vi "Apply Direction.vi"(8 "error in (no error)":errorcluster, 11 "Tool Rectangle in":refnum<class "Tool Rectangle.lvclass">) -> (0 "error out":errorcluster, 3 "Tool Rectangle out":refnum<class "Tool Rectangle.lvclass">)   [LabVIEW 2019, in "Tool Rectangle.lvclass"]
uses:
  Tool Rectangle.lvclass
  Settings/ObjectSettings/ObjectSettings.lvclass/ObjectSettings.ctl
  Settings/Rectangle Settings/Rectangle Settings.lvclass
  C:/Users/Albro/Documents/GitHub/AFM-Lithography/lvsrc/Classes/Settings/ObjectSettings/ObjectSettings.lvclass
  Settings/ObjectSettings/ObjectSettings.lvclass
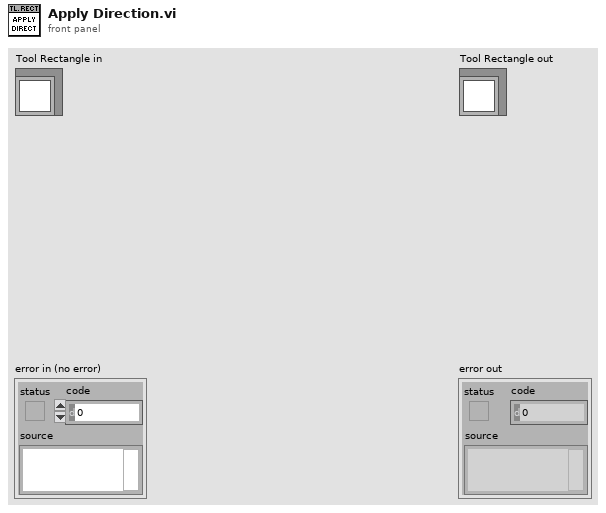
[diagram p1: front panel]
types:
  T1 = typedef "PathCommands.lvclass/Point.ctl" = cluster{"X":dbl, "Y":dbl}
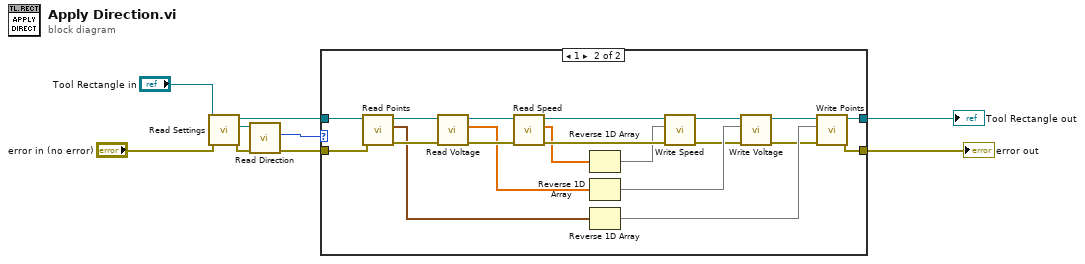
[diagram p0: block diagram]
diagram:
  n1 = call-dynamic "Read Settings.vi"("error in (no error)"="error in (no error)", "Tool Rectangle in"="Tool Rectangle in") -> ("error out"=w2:errorcluster, "Rectangle Settings.lvclass"=w6:refnum<class "Rectangle Settings.lvclass">, "Tool Rectangle out"=w5:refnum<class "Tool Rectangle.lvclass">)  [unwired: 7 in]
  n2 = call "Read Direction.vi"("error in (no error)"=w2, "ObjectSettings in"=w6) -> ("error out"=w3:errorcluster, "Direction"=w4:u16)  [unwired: 7 in, 1 out]
  n3 = case shown="1" w4 {
    tunnel: [w11 w16] -> w9
    tunnel: w5 -> [w11 w28]
    tunnel: w3 -> [w10 w27]
    tunnel: [w10 w15] -> w8
    frame 0, Default {
    }
    frame 1 {
      n4 = call-dynamic "Read Points.vi"("error in (no error)"=w27, "Tool Object in"=w28) -> ("error out"=w26:errorcluster, "Points"=w12:T1[], "Tool Object out"=w31:refnum<class "Tool Rectangle.lvclass">)  [unwired: 7 in]
      n5 = call-dynamic "Read Voltage.vi"("error in (no error)"=w26, "Tool Object in"=w31) -> ("error out"=w25:errorcluster, "Voltage"=w21:dbl[], "Tool Object out"=w30:refnum<class "Tool Rectangle.lvclass">)  [unwired: 7 in]
      n6 = call-dynamic "Read Speed.vi"("error in (no error)"=w25, "Tool Object in"=w30) -> ("error out"=w24:errorcluster, "Speed"=w23:dbl[], "Tool Object out"=w29:refnum<class "Tool Rectangle.lvclass">)  [unwired: 7 in]
      n7 = Reverse 1D Array(array=w23) -> (reversed array=w22:dbl[])
      n8 = Reverse 1D Array(array=w21) -> (reversed array=w19:dbl[])
      n9 = Reverse 1D Array(array=w12) -> (reversed array=w18:T1[])
      n10 = call-dynamic "Write Speed.vi"("error in (no error)"=w24, "Speed"=w22, "Tool Object in"=w29) -> ("error out"=w13:errorcluster, "Tool Object out"=w20:refnum<class "Tool Rectangle.lvclass">)  [unwired: 7 in]
      n11 = call-dynamic "Write Voltage.vi"("error in (no error)"=w13, "Voltage"=w19, "Tool Object in"=w20) -> ("error out"=w14:errorcluster, "Tool Object out"=w17:refnum<class "Tool Rectangle.lvclass">)  [unwired: 7 in]
      n12 = call-dynamic "Write Points.vi"("error in (no error)"=w14, "Points"=w18, "Tool Object in"=w17) -> ("error out"=w15:errorcluster, "Tool Object out"=w16:refnum<class "Tool Rectangle.lvclass">)  [unwired: 7 in]
    }
  }
  "error out" <- w8
  "Tool Rectangle out" <- w9
